vi "UMLEditor_FixXmlData.vi"(10 "XmlTemplateIn":string, 11 "xmlIn":string) -> (3 "XML OUt":string)   [LabVIEW 2012]
panel:
  in  "Multicolumn Listbox":i32(listbox)
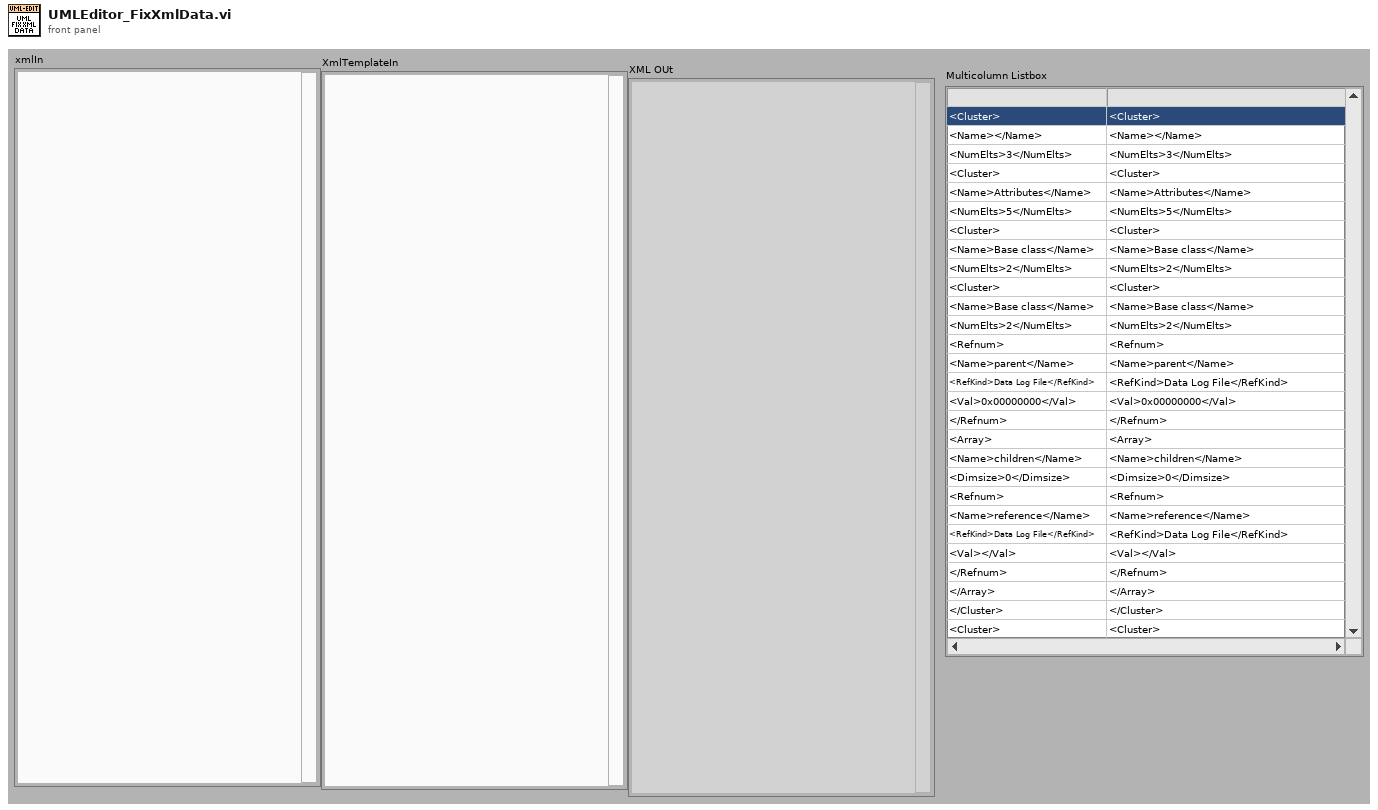
[diagram p1: front panel]
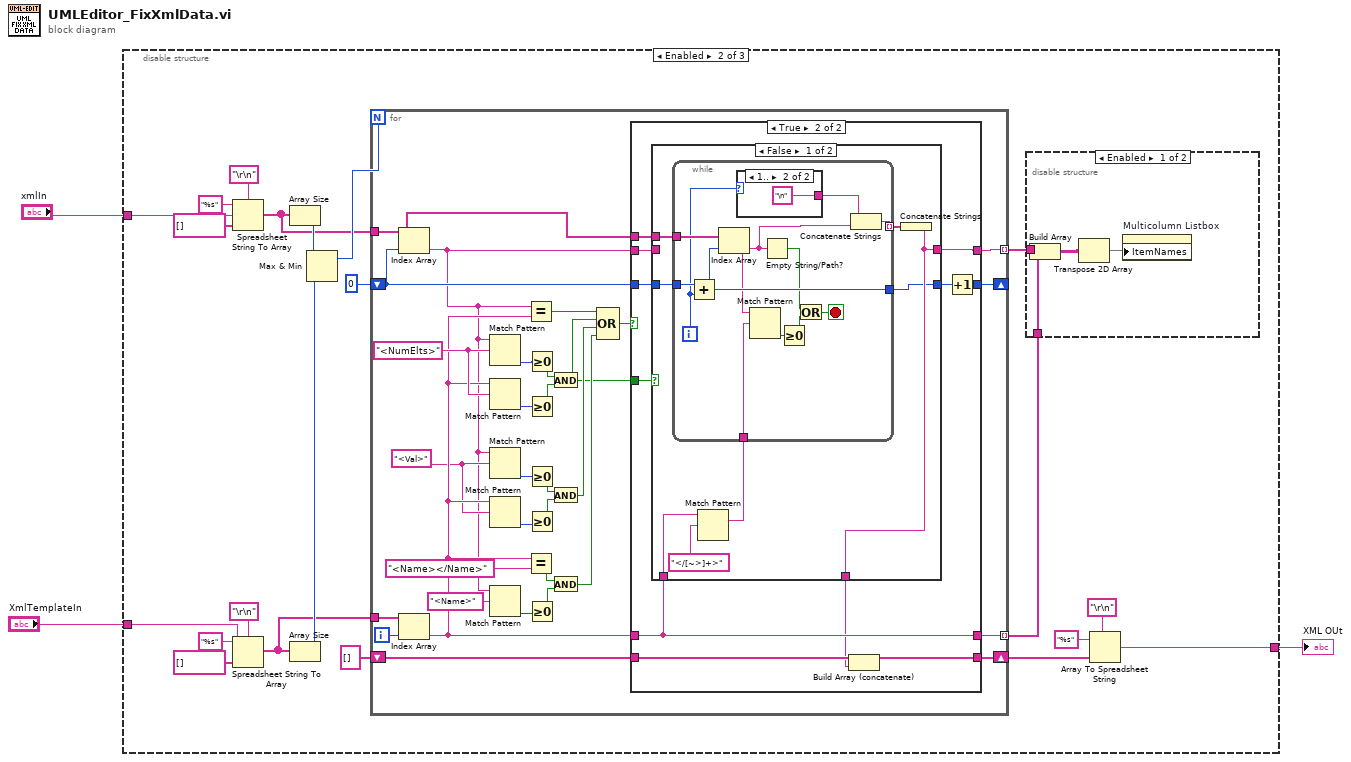
[diagram p0: block diagram]
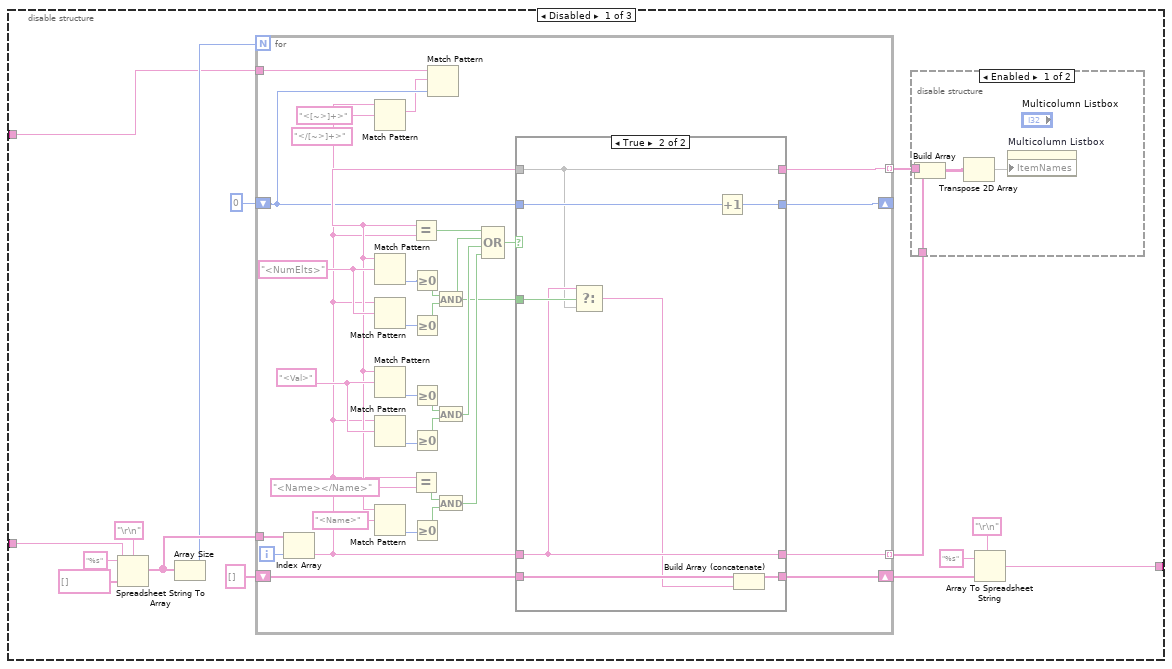
[diagram p2: hidden frame]
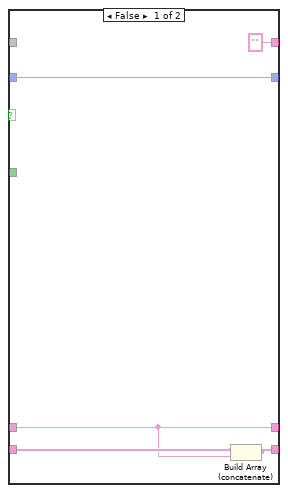
[diagram p4: hidden frame]
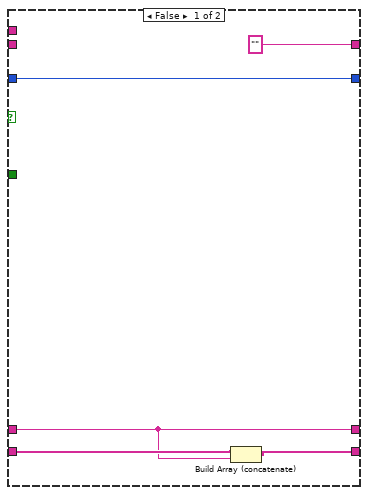
[diagram p6: hidden frame]
diagram:
  n1 = disable-structure shown="Enabled" {
    disable-tunnel: "xmlIn" -> [w4 w89 w165]
    disable-tunnel: "XmlTemplateIn" -> [w15 w82 _]
    disable-tunnel: [w6 w69 w165] -> w1
    frame Disabled {
      n2 = Spreadsheet String To Array(delimiter (Tab)="\r\n", format string="%s", spreadsheet string=w15, array type (2D Dbl)=string[] []) -> (array=w14:string[])
      n3 = Array Size(array=w14) -> (size(s)=w5:i32)
      n4 = for {
        N: w5 -> [_]
        tunnel: w14 -> [w55]
        shift-right: [w50] -> _
        shift-left: 0 -> [w24]
        tunnel: [w52] -> w12 mode=indexing
        tunnel: [w51] -> w11 mode=indexing
        shift-right: [w30] -> w9
        shift-left: string[] [] -> [w29]
        tunnel: w4 -> [w27]
        i -> [w53]
        (unwired) "</[~>]+>" ("regular expression")
        w37 = "<Val>" ("regular expression")
        w49 = "<NumElts>" ("regular expression")
        n5 = Index Array(array=w55, index=w53) -> (element=w26:string)
        n6 = Match Pattern(string=w26, regular expression="<[~>]+>") -> (match substring=w23:string)  [unwired: 4 out]
        n7 = Match Pattern(string=w26, regular expression=w49) -> (offset past match=w47:i32)  [unwired: 4 out]
        n8 = Match Pattern(string=w26, regular expression=w37) -> (offset past match=w39:i32)  [unwired: 4 out]
        n9 = Equal?(y=w26) -> (x=w31:string, x = y?=w54:bool)
        n10 = Match Pattern(string=w31, regular expression=w49) -> (offset past match=w48:i32)  [unwired: 4 out]
        n11 = Match Pattern(string=w31, regular expression=w37) -> (offset past match=w41:i32)  [unwired: 4 out]
        n12 = Match Pattern(string=w31, regular expression="<Name>") -> (offset past match=w35:i32)  [unwired: 4 out]
        n13 = Equal?(x=w26, y="<Name></Name>") -> (x = y?=w34:bool)
        n14 = Greater Or Equal To 0?(x=w48) -> (x >= 0?=w46:bool)
        n15 = Greater Or Equal To 0?(x=w47) -> (x >= 0?=w45:bool)
        n16 = Greater Or Equal To 0?(x=w41) -> (x >= 0?=w42:bool)
        n17 = Greater Or Equal To 0?(x=w39) -> (x >= 0?=w43:bool)
        n18 = Greater Or Equal To 0?(x=w35) -> (x >= 0?=w33:bool)
        n19 = Match Pattern(string=w27, regular expression=w23, offset (0)=w24) -> ()  [unwired: 4 out]
        n20 = And(x=w46, y=w45) -> (x .and. y?=w28:bool)
        n21 = And(x=w42, y=w43) -> (x .and. y?=w40:bool)
        n22 = And(x=w34, y=w33) -> (x .and. y?=w32:bool)
        n23 = Compound Arithmetic op=OR(w54, w28, w40, w32) -> (w44:bool)
        n24 = case shown="True" w44 {
          tunnel: w24 -> [w60 w68]
          tunnel: w31 -> [_ w62]
          tunnel: w26 -> [w56 w63]
          tunnel: ["" w62] -> w52
          tunnel: [w56 w63] -> w51
          tunnel: [w60 w67] -> w50
          tunnel: [w57 w66] -> w30
          tunnel: w29 -> [w58 w65]
          tunnel: w28 -> [_ w64]
          frame False {
            n25 = Build Array (concatenate)(w58, w56) -> (w57:string[])
          }
          frame True {
            n26 = Select(t=w63, s=w64, f=w62) -> (s? t:f=w61:string)
            n27 = Increment(x=w68) -> (x+1=w67:i32)
            n28 = Build Array (concatenate)(w65, w61) -> (w66:string[])
          }
        }
      }
      n29 = disable-structure shown="Enabled" {
        disable-tunnel: w12 -> [w22 _]
        disable-tunnel: w11 -> [w21 _]
        frame Enabled {
          n30 = Build Array(w22, w21) -> (w20:string[][])
          n31 = Transpose 2D Array(2D array=w20) -> (transposed array=w19:string[][])
          n32 = property on="Multicolumn Listbox" class="MCListbox (strict)"("ItemNames"=w19) -> ()  [unwired: 2 in, 2 out]
        }
        frame Disabled {
        }
      }
      n33 = Array To Spreadsheet String(delimiter (Tab)="\r\n", array=w9, 3:"%s" ("format string")) -> (spreadsheet string=w6:string)
    }
    frame Enabled {
      n34 = Spreadsheet String To Array(delimiter (Tab)="\r\n", format string="%s", spreadsheet string=w89, array type (2D Dbl)=string[] []) -> (array=w78:string[])
      n35 = Spreadsheet String To Array(delimiter (Tab)="\r\n", format string="%s", spreadsheet string=w82, array type (2D Dbl)=string[] []) -> (array=w77:string[])
      n36 = Array Size(array=w78) -> (size(s)=w81:i32)
      n37 = Array Size(array=w77) -> (size(s)=w80:i32)
      n38 = Max & Min(x=w81, y=w80) -> (max(x,y)=w79:i32)  [unwired: 1 out]
      n39 = for {
        N: w79 -> [_]
        tunnel: w78 -> [w94]
        tunnel: w77 -> [w124]
        shift-right: [w118] -> _
        shift-left: 0 -> [w121]
        tunnel: [w120] -> w75 mode=indexing
        tunnel: [w119] -> w74 mode=indexing
        shift-right: [w97] -> w72
        shift-left: string[] [] -> [w96]
        i -> [w122]
        w104 = "<Val>" ("regular expression")
        w117 = "<NumElts>" ("regular expression")
        n40 = Index Array(array=w94, index=w121) -> (element=w98:string)
        n41 = Index Array(array=w124, index=w122) -> (element=w106:string)
        n42 = Match Pattern(string=w98, regular expression=w117) -> (offset past match=w116:i32)  [unwired: 4 out]
        n43 = Match Pattern(string=w106, regular expression=w117) -> (offset past match=w115:i32)  [unwired: 4 out]
        n44 = Match Pattern(string=w98, regular expression=w104) -> (offset past match=w109:i32)  [unwired: 4 out]
        n45 = Match Pattern(string=w106, regular expression=w104) -> (offset past match=w107:i32)  [unwired: 4 out]
        n46 = Match Pattern(string=w98, regular expression="<Name>") -> (offset past match=w102:i32)  [unwired: 4 out]
        n47 = Equal?(x=w98, y=w106) -> (x = y?=w123:bool)
        n48 = Equal?(x=w106, y="<Name></Name>") -> (x = y?=w101:bool)
        n49 = Greater Or Equal To 0?(x=w116) -> (x >= 0?=w114:bool)
        n50 = Greater Or Equal To 0?(x=w115) -> (x >= 0?=w113:bool)
        n51 = Greater Or Equal To 0?(x=w109) -> (x >= 0?=w110:bool)
        n52 = Greater Or Equal To 0?(x=w107) -> (x >= 0?=w111:bool)
        n53 = Greater Or Equal To 0?(x=w102) -> (x >= 0?=w100:bool)
        n54 = And(x=w114, y=w113) -> (x .and. y?=w95:bool)
        n55 = And(x=w110, y=w111) -> (x .and. y?=w108:bool)
        n56 = And(x=w101, y=w100) -> (x .and. y?=w99:bool)
        n57 = Compound Arithmetic op=OR(w123, w95, w108, w99) -> (w112:bool)
        n58 = case shown="True" w112 {
          tunnel: w121 -> [w129 w134]
          tunnel: w98 -> [_ w137]
          tunnel: w106 -> [w125 w138]
          tunnel: ["" w133] -> w120
          tunnel: [w125 w138] -> w119
          tunnel: [w129 w130] -> w118
          tunnel: [w126 w140] -> w97
          tunnel: w96 -> [w127 w139]
          tunnel: w95 -> [_ w135]
          tunnel: w94 -> [_ w132]
          frame False {
            n59 = Build Array (concatenate)(w127, w125) -> (w126:string[])
          }
          frame True {
            n60 = case shown="False" w135 {
              tunnel: w138 -> [w148 w164]
              tunnel: w137 -> [_ w163]
              tunnel: [w142 w164] -> w136
              tunnel: w134 -> [w145 w162]
              tunnel: [w141 w162] -> w131
              tunnel: [w142 w163] -> w133
              tunnel: w132 -> [w146 _]
              frame False {
                n61 = Match Pattern(string=w148, regular expression="</[~>]+>") -> (match substring=w144:string)  [unwired: 4 out]
                n62 = while {
                  tunnel: w146 -> [w160]
                  tunnel: w145 -> [w159]
                  tunnel: [w158] -> w141
                  tunnel: w144 -> [w157]
                  tunnel: [w151] -> w143 mode=indexing
                  i -> [w150]
                  stop <- w153 stop-if-true
                  n63 = Add(x=w159, y=w150) -> (x+y=w158:i32)
                  n64 = Index Array(array=w160, index=w158) -> (element=w152:string)
                  n65 = case shown="1.." w150 {
                    tunnel: [_ "\n" ("delimiter (Tab)")] -> w149
                    frame 0, Default {
                    }
                    frame 1.. {
                    }
                  }
                  n66 = Match Pattern(string=w152, regular expression=w157) -> (offset past match=w156:i32)  [unwired: 4 out]
                  n67 = Empty String/Path?(string/path=w152) -> (empty?=w154:bool)
                  n68 = Greater Or Equal To 0?(x=w156) -> (x >= 0?=w155:bool)
                  n69 = Or(x=w154, y=w155) -> (x .or. y?=w153:bool)
                  n70 = Concatenate Strings(w149, w152) -> (w151:string)
                }
                n71 = Concatenate Strings(w143) -> (w142:string)
              }
              frame True {
              }
            }
            n72 = Build Array (concatenate)(w139, w136) -> (w140:string[])
            n73 = Increment(x=w131) -> (x+1=w130:i32)
          }
        }
      }
      n74 = disable-structure shown="Enabled" {
        disable-tunnel: w75 -> [w93 _]
        disable-tunnel: w74 -> [w92 _]
        frame Enabled {
          n75 = Build Array(w93, w92) -> (w91:string[][])
          n76 = Transpose 2D Array(2D array=w91) -> (transposed array=w90:string[][])
          n77 = property on="Multicolumn Listbox" class="MCListbox (strict)"("ItemNames"=w90) -> ()  [unwired: 2 in, 2 out]
        }
        frame Disabled {
        }
      }
      n78 = Array To Spreadsheet String(delimiter (Tab)="\r\n", array=w72, 3:"%s" ("format string")) -> (spreadsheet string=w69:string)
    }
    frame Disabled {
    }
  }
  "XML OUt" <- w1
